vi "getState0.vi"(8 "error in (no error)":errorcluster, 11 "ZTAAC in":refnum<class "ZTAAC.lvclass">) -> (0 "error out":errorcluster, 2 "State 0 in DOF":dbl[](array[numeric]), 3 "ZTAAC out":refnum<class "ZTAAC.lvclass">)   [LabVIEW 2016, in "ZTAAC.lvclass"]
doc: "Get the state 0 in degree of freedom (DOF)."
uses:
  ZTAAC.lvclass
  ZTAAC.lvclass/ZTAAC.ctl
  OptCtrl/OptCtrl.lvclass
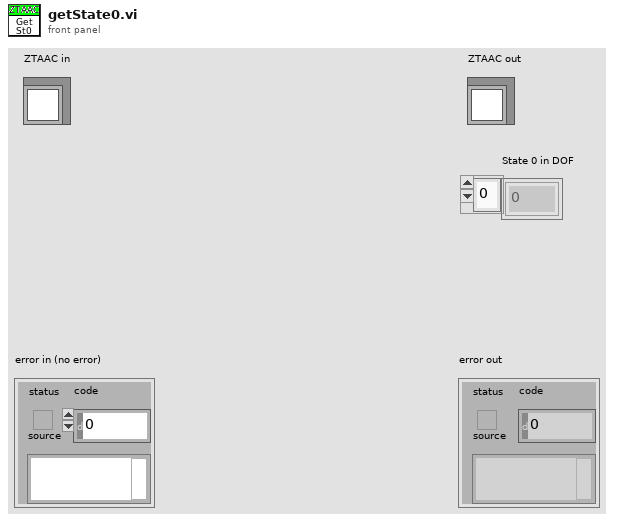
[diagram p1: front panel]
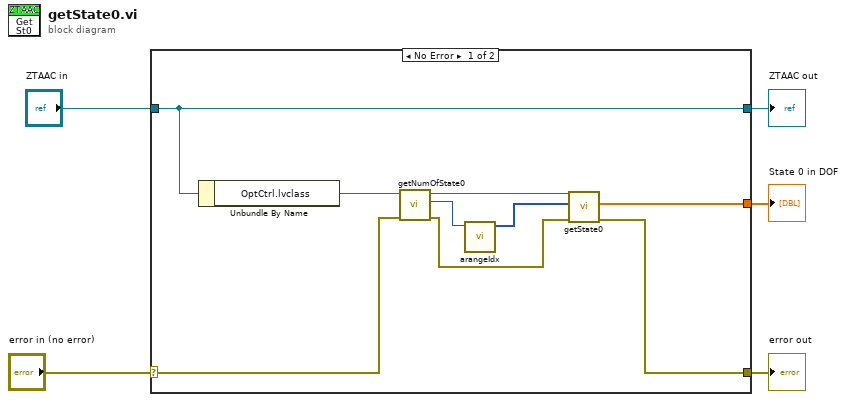
[diagram p0: block diagram]
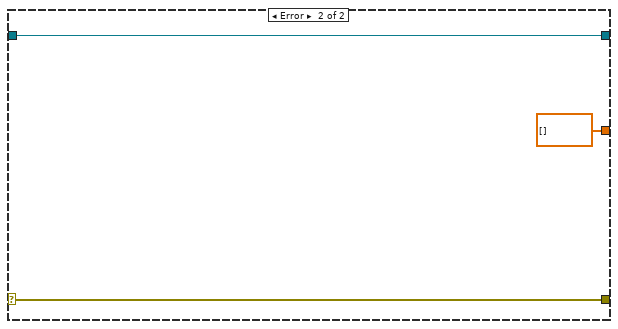
[diagram p2: hidden frame]
diagram:
  n1 = case shown="No Error" "error in (no error)" {
    selector: "error in (no error)" -> [w8 w17]
    tunnel: [w6 w17] -> w4
    tunnel: [w14 w16] -> w2
    tunnel: "ZTAAC in" -> [w14 w16]
    tunnel: [w9 dbl[] [] ("State 0 in DOF")] -> w1
    frame No Error {
      n2 = Unbundle By Name(w14) -> ("OptCtrl.lvclass"=w13:refnum<class "OptCtrl.lvclass">)
      n3 = call "getNumOfState0.vi"("error in (no error)"=w8, "OptCtrl in"=w13) -> ("error out"=w7:errorcluster, "Num of State 0"=w12:i32, "OptCtrl out"=w11:refnum<class "OptCtrl.lvclass">)  [unwired: 7 in]
      n4 = call "arangeIdx.vi"("Number"=w12) -> ("Idx Array"=w10:i32[])  [unwired: 10 in]
      n5 = call "getState0.vi"("error in (no error)"=w7, "dofIdx"=w10, "OptCtrl in"=w11) -> ("error out"=w6:errorcluster, "State 0 in DOF"=w9:dbl[])  [unwired: 6 in, 1 out]
    }
    frame Error {
    }
  }
  "error out" <- w4
  "ZTAAC out" <- w2
  "State 0 in DOF" <- w1
